vi "NewVI.vi"(1 "Option":u32, 2 "Path":path, 3 "Ref":refnum<vi>) -> (0 "VI":refnum<vi>)   [LabVIEW 2014]
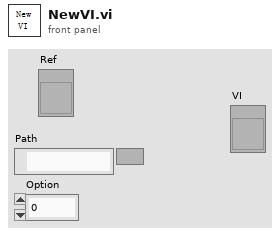
[diagram p1: front panel]
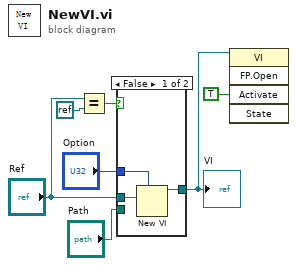
[diagram p0: block diagram]
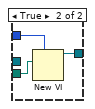
[diagram p2: hidden frame]
diagram:
  n1 = Equal?(x="Ref", y=refnum<k0> refnum) -> (x = y?=w6:bool)
  n2 = case shown="False" w6 {
    tunnel: "Ref" -> [w10 _]
    tunnel: "Option" -> [w9 w12]
    tunnel: [w8 w11] -> w2
    tunnel: "Path" -> [_ w13]
    frame False {
      n3 = New VI(7:w9, 10:w10) -> (3:w8:refnum<vi>)  [unwired: 5 in, 1 out]
    }
    frame True {
      n4 = New VI(7:w12, 10:w13) -> (3:w11:refnum<vi>)  [unwired: 5 in, 1 out]
    }
  }
  "VI" <- w2
  n5 = invoke class="VI" method="FP.Open"(reference=w2, "Activate"=TRUE ("Activate?")) -> ()  [unwired: 3 in, 5 out]
